vi "TurnAimForward.vi"() -> (3 "RobotDriveDevRef":T1={"DevStatus"={"status"=FALSE, "code"=0, "source"=""}, "Motors[]"=[], "Square Inputs"=FALSE, "Max Output"=1.0})   [LabVIEW 2016]
uses:
  <vilib>/Rock Robotics/WPI/RobotDrive/WPI_RobotDriveArcadeDrive_Standard(NoSaturation).vi
  Robot Global Data.vi
  <vilib>/Rock Robotics/SystemInterfaces/DIO/FPGA_DIOPWMChannel.ctl
  <vilib>/Rock Robotics/WPI/PWM/WPI_PWMDeadband.ctl
  <vilib>/Rock Robotics/WPI/MotorControl/WPI_MotorControlType.ctl
  <vilib>/Rock Robotics/WPI/MotorControl/WPI_MotorControlDeviceRef.ctl
  <vilib>/Rock Robotics/WPI/RobotDrive/WPI_RobotDriveDevRef.ctl
panel:
  in  "Angle":dbl
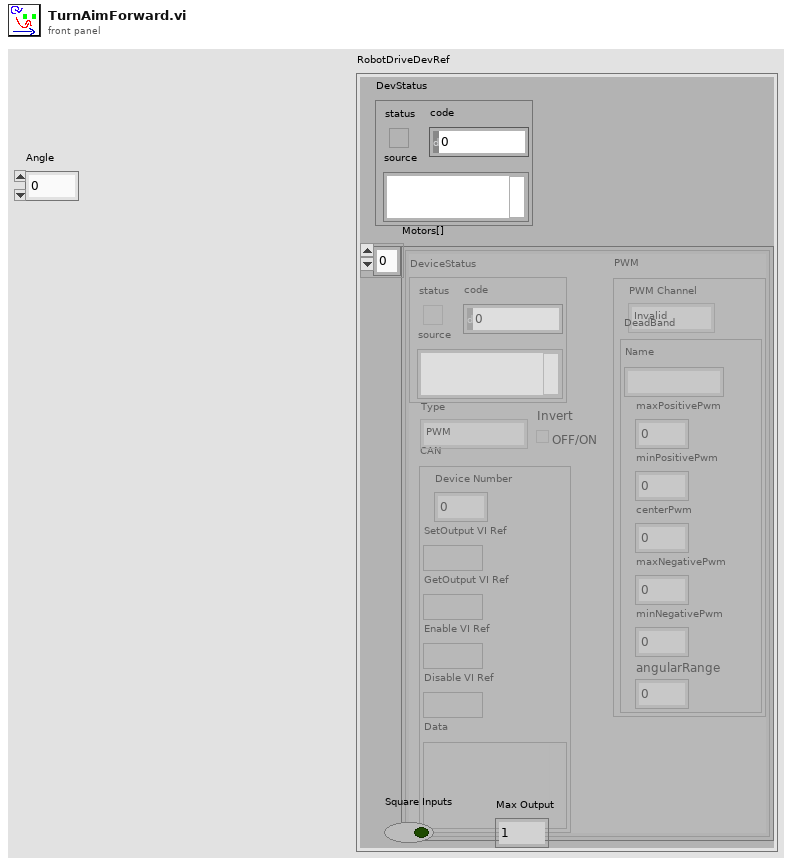
[diagram p1: front panel]
types:
  T1 = typedef "WPI_RobotDriveDevRef.ctl" = cluster{"DevStatus":errorcluster, "Motors[]":T2[], "Square Inputs":bool, "Max Output":dbl}
  T2 = typedef "WPI_MotorControlDeviceRef.ctl" = cluster{"DeviceStatus":errorcluster, "Type":T3, "PWM":cluster{"PWM Channel":T4, "DeadBand":T5}, "CAN":cluster{"Device Number":u8, "SetOutput VI Ref":variant, "GetOutput VI Ref":variant, "Enable VI Ref":variant, "Disable VI Ref":variant, "Data":variant}, "Invert":bool}
  T3 = typedef "WPI_MotorControlType.ctl" = enum16{"PWM", "CAN"}
  T4 = typedef "FPGA_DIOPWMChannel.ctl" = enum8{"PWM 0", "PWM 1", "PWM 2", "PWM 3", "PWM 4", "PWM 5", "PWM 6", "PWM 7", "PWM 8", "PWM 9", "PWM MXP 0", "PWM MXP 1", "PWM MXP 2", "PWM MXP 3", "PWM MXP 4", "PWM MXP 5", "PWM MXP 6", "PWM MXP 7", "PWM MXP 8", "PWM MXP 9", "Invalid"}
  T5 = typedef "WPI_PWMDeadband.ctl" = cluster{"Name":string, "maxPositivePwm":i32, "minPositivePwm":i32, "centerPwm":i32, "maxNegativePwm":i32, "minNegativePwm":i32, "angularRange":u16}
  T6 = cluster{"Lower X":dbl, "Lower Y":dbl, "Upper X":dbl, "Upper Y":dbl, "Lower Limit":dbl, "Upper Limit":dbl}
  T7 = cluster{"Target?":bool, "Angle":dbl, "Distance":dbl}
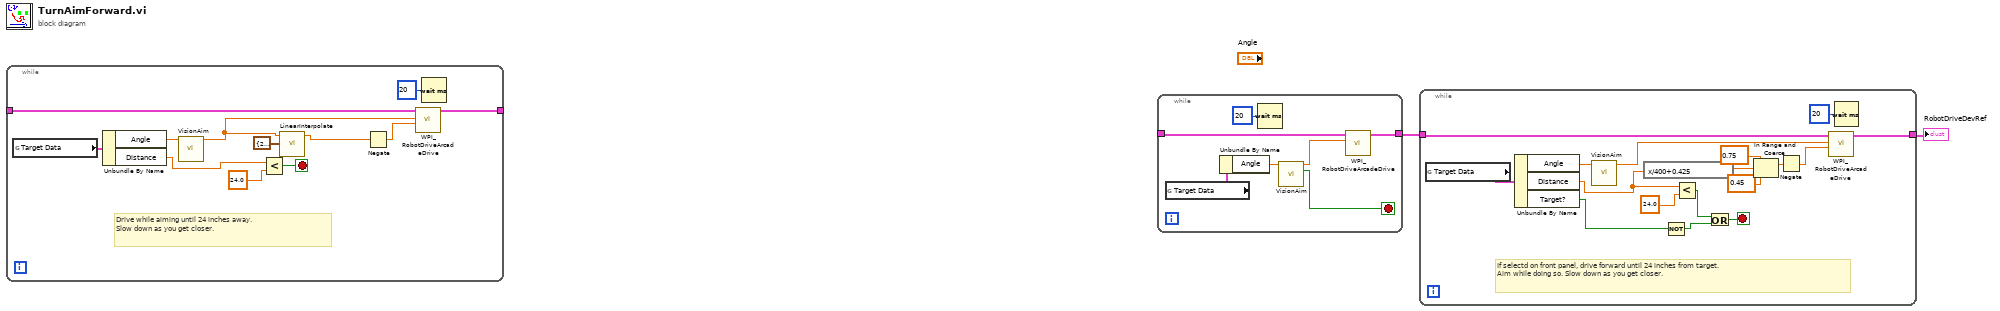
[diagram p0: block diagram]
diagram:
  n1 = while {
    tunnel: _ -> [w14]
    tunnel: [w13] -> _
    stop <- w11 stop-if-true
    # "Drive while aiming until 24 inches away.\nSlow down as you get closer."
    n2 = global read "Robot Global Data.vi" "Target Data"() -> (w8:T7)
    n3 = Unbundle By Name(w8) -> ("Angle"=w7:dbl, "Distance"=w6:dbl)
    n4 = call "VisionAim.vi"("Angle"=w7) -> ("Turn Amount"=w4:dbl)  [unwired: 9 in, 1 out]
    n5 = Less?(x=w6, y=24.0) -> (x < y?=w11:bool)
    n6 = call "LinearInterpolate.vi"("Config"=T6 {"Lower X"=24.0, "Lower Y"=0.48, "Upper X"=65.0, "Upper Y"=0.8, "Lower Limit"=0.45, "Upper Limit"=0.75}, "Value"=w4) -> ("Ouput"=w3:dbl)  [unwired: 9 in]
    n7 = Negate(x=w3) -> (-x=w9:dbl)
    n8 = call-poly <vilib>:"WPI_RobotDriveArcadeDrive.vi"("Y axis value"=w9, "X axis value"=w4, "RobotDriveDevRef"=w14) -> ("RobotDriveDevRef"=w13:T1)  [unwired: 6 in, 2 out]
    n9 = Wait (ms)(milliseconds to wait=u32 20) -> ()  [unwired: 1 out]
  }
  n10 = while {
    tunnel: _ -> [w21]
    tunnel: [w17] -> w2
    stop <- w19 stop-if-true
    n11 = global read "Robot Global Data.vi" "Target Data"() -> (w16:T7)
    n12 = Unbundle By Name(w16) -> ("Angle"=w15:dbl)
    n13 = Wait (ms)(milliseconds to wait=u32 20) -> ()  [unwired: 1 out]
    n14 = call "VisionAim.vi"("Angle"=w15) -> ("In Range"=w19:bool, "Turn Amount"=w20:dbl)  [unwired: 9 in]
    n15 = call-poly <vilib>:"WPI_RobotDriveArcadeDrive.vi"("X axis value"=w20, "RobotDriveDevRef"=w21) -> ("RobotDriveDevRef"=w17:T1)  [unwired: 7 in, 2 out]
  }
  n16 = while {
    tunnel: w2 -> [w37]
    tunnel: [w36] -> w1
    stop <- w24 stop-if-true
    # "If selectd on front panel, drive forward until 24 inches from target.\nAim while doing so. Slow down as you get closer."
    n17 = global read "Robot Global Data.vi" "Target Data"() -> (w28:T7)
    n18 = Unbundle By Name(w28) -> ("Angle"=w27:dbl, "Distance"=w26:dbl, "Target?"=w22:bool)
    n19 = call "VisionAim.vi"("Angle"=w27) -> ("Turn Amount"=w38:dbl)  [unwired: 9 in, 1 out]
    n20 = expression code="x/400+0.425"(w26) -> (w33:dbl)
    n21 = Not(x=w22) -> (.not. x?=w23:bool)
    n22 = Less?(x=w26, y=24.0) -> (x < y?=w25:bool)
    n23 = Or(x=w25, y=w23) -> (x .or. y?=w24:bool)
    n24 = In Range and Coerce(upper limit=0.75, x=w33, lower limit=0.45) -> (coerced(x)=w30:dbl)  [unwired: 1 out]
    n25 = Negate(x=w30) -> (-x=w29:dbl)
    n26 = call-poly <vilib>:"WPI_RobotDriveArcadeDrive.vi"("Y axis value"=w29, "X axis value"=w38, "RobotDriveDevRef"=w37) -> ("RobotDriveDevRef"=w36:T1)  [unwired: 6 in, 2 out]
    n27 = Wait (ms)(milliseconds to wait=u32 20) -> ()  [unwired: 1 out]
  }
  "RobotDriveDevRef" <- w1
